vi "Untitled 2.vi"() -> ()   [LabVIEW 2011]
uses:
  <vilib>/LabVIEW Interface for Arduino/Type Defs/Pin Mode.ctl
  <vilib>/LabVIEW Interface for Arduino/LabVIEW Interface for Arduino.lvlib
panel:
  out "PWM Pins":u8[](array[numeric])
types:
  T1 = typedef "LabVIEW Interface for Arduino.lvlib/Pin Mode.ctl" = enum8{"Input", "Output"}
  T2 = typedef "LabVIEW Interface for Arduino.lvlib/Arduino Resource.ctl" = cluster{"VISA resource":refnum<visa-resource-name>, "Board Type":T3, "Connection Type":enum8{"USB / Serial"}, "Bytes Per Packet (15)":u8}
  T3 = typedef "LabVIEW Interface for Arduino.lvlib/Board Type.ctl" = enum16{"Uno", "Dimuelanove w/Atmega 328", "Mega 2560"}
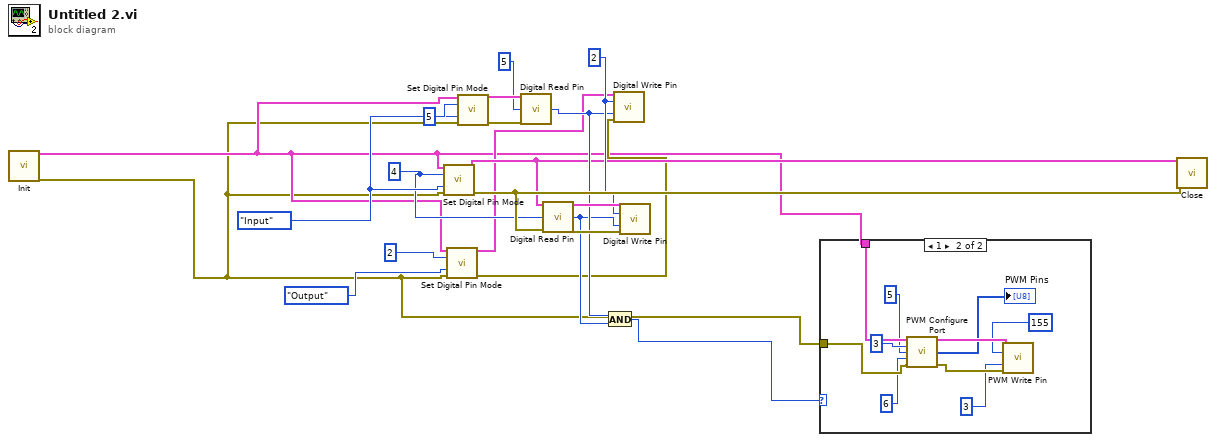
[diagram p0: block diagram]
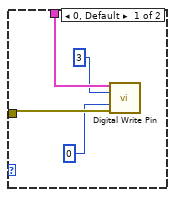
[diagram p2: hidden frame]
diagram:
  w9 = u8 2 ("Digital I/O Pin (0)")
  w18 = Pin_Mode."Input" ("Pin Mode (Input)")
  w12 = u8 4 ("Digital I/O Pin")
  n1 = call <vilib>:"Init.vi"() -> ("Arduino Resource"=w2:T2, "error out"=w1:errorcluster)  [unwired: 18 in]
  n2 = call <vilib>:"Set Digital Pin Mode.vi"("Arduino Resource"=w2, "Digital I/O Pin"=w12, "Pin Mode (Input)"=w18, "error in"=w1) -> ("Arduino Resource"=w6:T2, "error out"=w13:errorcluster)  [unwired: 10 in]
  n3 = call <vilib>:"Set Digital Pin Mode.vi"("Arduino Resource"=w2, "Digital I/O Pin"=u8 2, "Pin Mode (Input)"=Pin_Mode."Output", "error in"=w1) -> ("Arduino Resource"=w5:T2, "error out"=w4:errorcluster)  [unwired: 10 in]
  n4 = call <vilib>:"Set Digital Pin Mode.vi"("Arduino Resource"=w2, "Digital I/O Pin"=u8 5, "Pin Mode (Input)"=w18, "error in"=w1) -> ("Arduino Resource"=w15:T2, "error out"=w16:errorcluster)  [unwired: 10 in]
  n5 = call <vilib>:"Digital Read Pin.vi"("Arduino Resource"=w15, "Digital I/O Pin (0)"=u8 5, "error in"=w16) -> ("Value"=w8:u8)  [unwired: 10 in, 2 out]
  n6 = call <vilib>:"Digital Read Pin.vi"("Arduino Resource"=w6, "Digital I/O Pin (0)"=w12, "error in"=w13) -> ("Arduino Resource"=w11:T2, "Value"=w7:u8, "error out"=w10:errorcluster)  [unwired: 10 in]
  n7 = And(x=w8, y=w7) -> (x .and. y?=w3:u8)
  n8 = call <vilib>:"Digital Write Pin.vi"("Arduino Resource"=w5, "Digital I/O Pin (0)"=w9, "Value (0)"=w8, "error in"=w4) -> ()  [unwired: 10 in, 2 out]
  n9 = call <vilib>:"Digital Write Pin.vi"("Arduino Resource"=w11, "Digital I/O Pin (0)"=w9, "Value (0)"=w7, "error in"=w10) -> ()  [unwired: 10 in, 2 out]
  n10 = case shown="1" w3 {
    tunnel: w2 -> [w24 w30]
    tunnel: w1 -> [w23 w29]
    frame 0, Default {
      n11 = call <vilib>:"Digital Write Pin.vi"("Arduino Resource"=w24, "Digital I/O Pin (0)"=u8 3, "Value (0)"=u8 0, "error in"=w23) -> ()  [unwired: 10 in, 2 out]
    }
    frame 1 {
      n12 = call <vilib>:"PWM Configure Port.vi"("Arduino Resource"=w30, "PWM Pin (3)"=u8 3, "PWM Pin (5)"=u8 5, "PWM Pin (6)"=u8 6, "error in"=w29) -> ("Arduino Resource"=w34:T2, "PWM Pins"=→"PWM Pins":u8[], "error out"=w33:errorcluster)  [unwired: 8 in]
      n13 = call <vilib>:"PWM Write Pin.vi"("Arduino Resource"=w34, "Duty Cycle (0 - 255)"=u8 155, "PWM Pin (3)"=u8 3, "error in"=w33) -> ()  [unwired: 10 in, 2 out]
    }
  }
  n14 = call <vilib>:"Close.vi"("Arduino Resource"=w6, "error in"=w13) -> ()  [unwired: 13 in, 1 out]
